vi "Send LCD Data.vi"() -> ()   [LabVIEW 2013]
uses:
  <vilib>/rvi/interface/nirviMethod/nirviMethod.xnode
  <vilib>/rvi/errors/niLvFpgaMergeErrorWithErrorCode.vi
  <vilib>/rvi/interface/nirviReadWriteControl/nirviReadWriteControl.xnode
  <vilib>/rvi/interface/Simulation/niFpgaSimulationCallBeginRW.vi
  <vilib>/rvi/errors/niLvFpgaAdjustHostInterfaceError.vi
  <vilib>/rvi/interface/nirviOpenFPGA/nirviOpenFPGA.xnode
  LEDMatrix_2/FPGA Bitfiles/LEDMatrix2_FPGATarget_LCDSPI_P5VCD-4LKxw.lvbitx
  LEDMatrix_2/LCD SPI.vi
  <vilib>/FPGAPlugInAG/Dynamic/niLvFpga_StartFifo_Dynamic.vi
  <vilib>/FPGAPlugInAG/Dynamic/niLvFpga_StopFifo_Dynamic.vi
  <vilib>/FPGAPlugInAG/Dynamic/niLvFpga_ConfigureFifo_Dynamic.vi
  Cluser.ctl
panel:
  in  "stop":bool
  in  "Tab Control":T1(tab)
  in  "Display Rectangle":bool
  in  "Cluster":T2={"x start"=47, "x end"=79, "y start"=47, "y end"=111, "Color Up"=255, "Color Lower"=255}
  in  "BMP Name":string="stars.bmp"
  in  "Display Image":bool
  out "Accel X":i16
  out "Accel Y":i16
  out "Accel Z":i16
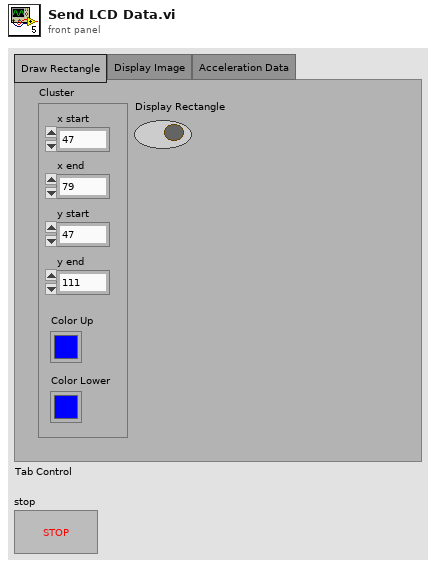
[diagram p1: front panel]
types:
  T1 = enum32{"Draw Rectangle", "Display Image", "Acceleration Data"}
  T2 = typedef "Cluser.ctl" = cluster{"x start":u16, "x end":u16, "y start":u16, "y end":u16, "Color Up":u32, "Color Lower":u32}
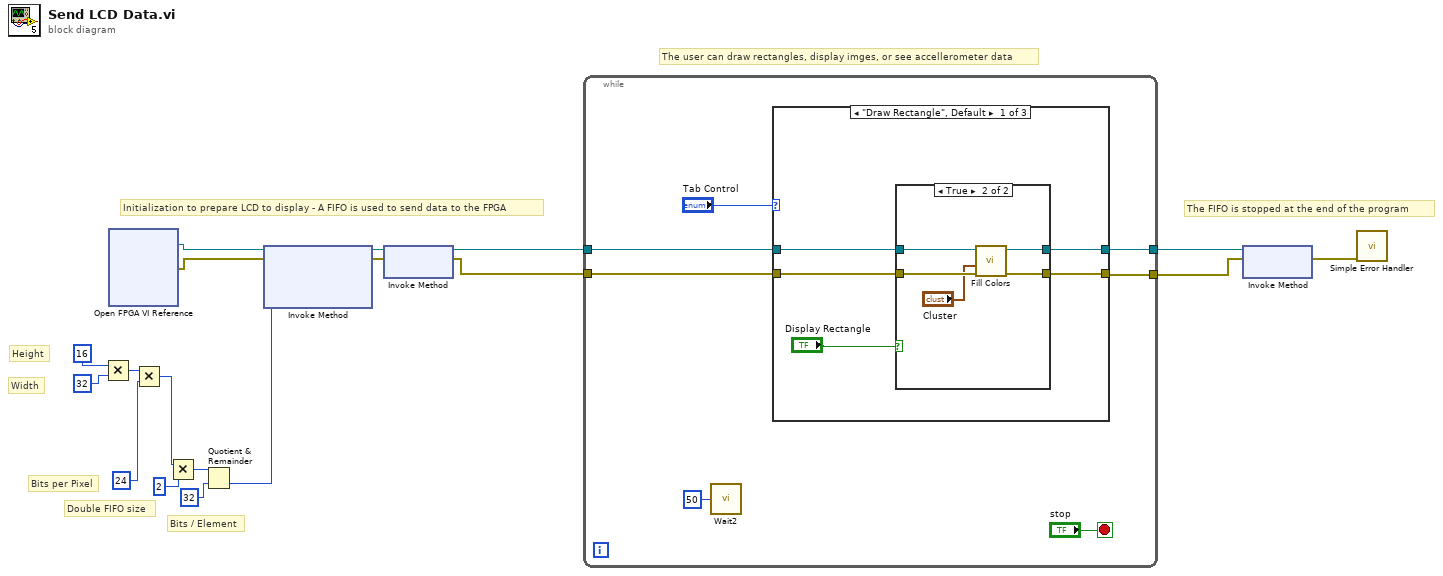
[diagram p0: block diagram]
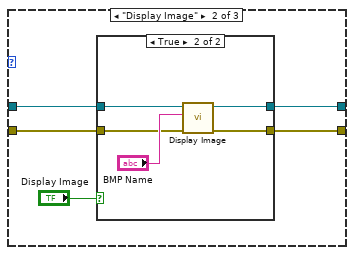
[diagram p3: hidden frame]
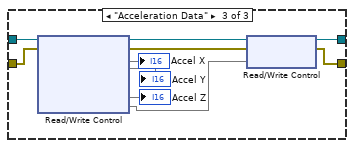
[diagram p5: hidden frame]
diagram:
  # "Bits / Element"
  # "Double FIFO size"
  # "Bits per Pixel"
  # "Width"
  # "Height"
  # "The FIFO is stopped at the end of the program"
  # "The user can draw rectangles, display imges, or see accellerometer data"
  # "Initialization to prepare LCD to display - A FIFO is used to send data to the FPGA"
  n1 = Multiply(x=u32 16 ("Requested Depth"), y=u32 32 ("Requested Depth")) -> (x*y=w9:u32)
  n2 = xnode "Open FPGA VI Reference"() -> ("FPGA VI Reference Out"=w13:refnum<k20>, "error out"=w12:errorcluster)  [unwired: 2 in]
  n3 = Multiply(x=w9, y=u32 24 ("Requested Depth")) -> (x*y=w7:u32)
  n4 = Multiply(x=w7, y=u32 2 ("Requested Depth")) -> (x*y=w5:u32)
  n5 = Quotient & Remainder(x=w5, y=u32 32 ("Requested Depth")) -> (floor(x/y)=w3:u32)  [unwired: 1 out]
  n6 = xnode "Invoke Method"("FPGA VI Reference In"=w13, "error in"=w12, "Requested Depth"=w3) -> ("FPGA VI Reference Out"=w18:refnum<k20>, "error out"=w17:errorcluster)  [unwired: 1 out]
  n7 = xnode "Invoke Method"("FPGA VI Reference In"=w18, "error in"=w17) -> ("FPGA VI Reference Out"=w2:refnum<k20>, "error out"=w1:errorcluster)
  n8 = while {
    tunnel: w2 -> [w24]
    tunnel: w1 -> [w23]
    tunnel: [w22] -> w15
    tunnel: [w21] -> w14
    stop <- "stop" stop-if-true
    n9 = call "Wait2"("Count(mSec)"=u32 50) -> ()  [unwired: 1 out]
    n10 = case shown="\"Draw Rectangle\", Default" "Tab Control" {
      tunnel: w24 -> [w30 w40 w59]
      tunnel: w23 -> [w29 w39 w58]
      tunnel: [w28 w42 w57] -> w22
      tunnel: [w27 w41 w56] -> w21
      frame "Draw Rectangle", Default {
        n11 = case shown="True" "Display Rectangle" {
          tunnel: [w32 w37] -> w28
          tunnel: [w31 w36] -> w27
          tunnel: w30 -> [w32 w35]
          tunnel: w29 -> [w31 w34]
          frame False {
          }
          frame True {
            n12 = call "Fill Colors.vi"("error in (no error)"=w34, "Cluster"="Cluster", "Refnum in"=w35) -> ("error out"=w36:errorcluster, "Refnum out"=w37:refnum<k20>)  [unwired: 6 in, 1 out]
          }
        }
      }
      frame "Display Image" {
        n13 = case shown="True" "Display Image" {
          tunnel: [w44 w48] -> w42
          tunnel: [w43 w47] -> w41
          tunnel: w40 -> [w44 w46]
          tunnel: w39 -> [w43 w45]
          frame False {
          }
          frame True {
            n14 = call "Display Image.vi"("error in (no error)"=w45, "path to BMP file on myRio local filesystem"="BMP Name", "Refnum in"=w46) -> ("error out"=w47:errorcluster, "Refnum out"=w48:refnum<k20>)  [unwired: 4 in, 3 out]
          }
        }
      }
      frame "Acceleration Data" {
        n15 = xnode "Read/Write Control"("FPGA VI Reference In"=w59, "error in"=w58) -> ("FPGA VI Reference Out"=w55:refnum<k20>, "error out"=w54:errorcluster, "AccelerationX"=→"Accel X", "AccelerationY"=→"Accel Y", "AccelerationZ"=→"Accel Z", "S5/DIO0"=w50)
        n16 = xnode "Read/Write Control"("FPGA VI Reference In"=w55, "error in"=w54, "LED/DIO9"=w50) -> ("FPGA VI Reference Out"=w57:refnum<k20>, "error out"=w56:errorcluster)
      }
    }
  }
  n17 = xnode "Invoke Method"("FPGA VI Reference In"=w15, "error in"=w14) -> ("error out"=w16:errorcluster)  [unwired: 1 out]
  n18 = call <vilib>:"Simple Error Handler.vi"("error in (no error)"=w16) -> ()  [unwired: 4 in, 5 out]
